vi "execute.vi"(8 "error in (no error)":errorcluster, 9 "image assembler in":refnum<class "GenericComponent.lvclass">, 10 "trajectory in":refnum<class "GenericComponent.lvclass">, 11 "AdapterMH111103TrajectoryToImageAssembler in":refnum<class "AdapterMH111103TrajectoryToImageAssembler.lvclass">) -> (0 "error out":errorcluster, 1 "image assembler out":refnum<class "GenericComponent.lvclass">, 2 "trajectory out":refnum<class "GenericComponent.lvclass">, 3 "AdapterMH111103TrajectoryToImageAssembler out":refnum<class "AdapterMH111103TrajectoryToImageAssembler.lvclass">)   [LabVIEW 2010, in "AdapterMH111103TrajectoryToImageAssembler.lvclass"]
uses:
  AdapterMH111103TrajectoryToImageAssembler.lvclass
  common/classes/GenericComponent/GenericComponent/GenericComponent.lvclass
  ImageAssembler/ImageAssemblerDL090211Frame/ImageAssemblerDL090211Frame/ImageAssemblerDL090211Frame.lvclass
  Trajectory/TrajectoryMG100122AODFrameScan/TrajectoryMG100122AODFrameScan/TrajectoryMG100122AODFrameScan.lvclass
  common/classes/Box/Box/Box.lvclass
  common/classes/SpaceVector/SpaceVector/SpaceVector.lvclass
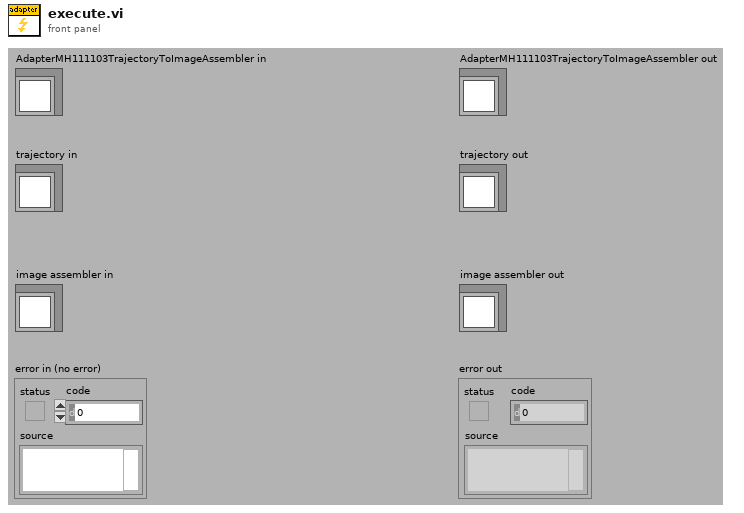
[diagram p1: front panel]
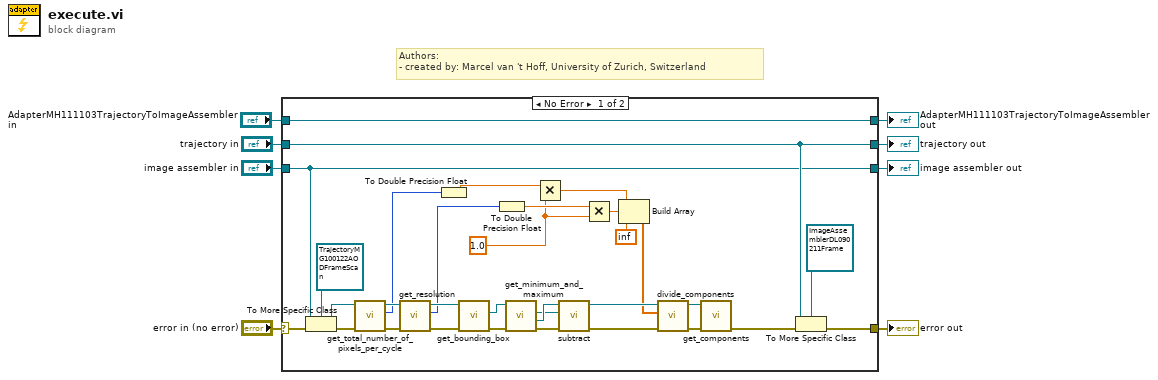
[diagram p0: block diagram]
diagram:
  # "Authors: \n- created by: Marcel van 't Hoff, University of Zurich, Switzerland"
  n1 = case shown="No Error" "error in (no error)" {
    selector: "error in (no error)" -> [w20 w43]
    tunnel: [w19 w43] -> w4
    tunnel: [w40 w44] -> w1
    tunnel: "AdapterMH111103TrajectoryToImageAssembler in" -> [w40 w44]
    tunnel: [w37 w42] -> w2
    tunnel: "trajectory in" -> [w37 w42]
    tunnel: [w9 w41] -> w3
    tunnel: "image assembler in" -> [w9 w41]
    frame No Error {
      w11 = 1.0
      n2 = To More Specific Class(target class=refnum<class "TrajectoryMG100122AODFrameScan.lvclass"> refnum ("TrajectoryMG100122AODFrameScan.lvclass"), reference=w9, error in=w20) -> (specific class reference=w36:refnum<class "TrajectoryMG100122AODFrameScan.lvclass">, error out=w33:errorcluster)
      n3 = call-dynamic "get_total_number_of_pixels_per_cycle.vi"("error in (no error)"=w33, "TrajectoryMG100122AODFrameScan in"=w36) -> ("error out"=w34:errorcluster, "total number of pixels per cycle"=w13:i32, "TrajectoryMG100122AODFrameScan out"=w35:refnum<class "TrajectoryMG100122AODFrameScan.lvclass">)  [unwired: 7 in]
      n4 = call-dynamic "get_resolution.vi"("error in (no error)"=w34, "TrajectoryMG100122AODFrameScan in"=w35) -> ("error out"=w22:errorcluster, "x resolution"=w12:i32, "TrajectoryMG100122AODFrameScan out"=w23:refnum<class "TrajectoryMG100122AODFrameScan.lvclass">)  [unwired: 6 in, 1 out]
      n5 = To Double Precision Float(number=w13) -> (double precision float=w15:dbl)
      n6 = call-dynamic "get_bounding_box.vi"("error in (no error)"=w22, "GenericTrajectory in"=w23) -> ("error out"=w24:errorcluster, "Box.lvclass"=w25:refnum<class "Box.lvclass">)  [unwired: 7 in, 1 out]
      n7 = To Double Precision Float(number=w12) -> (double precision float=w16:dbl)
      n8 = call "get_minimum_and_maximum.vi"("error in (no error)"=w24, "Box in"=w25) -> ("error out"=w26:errorcluster, "maximum"=w28:refnum<class "SpaceVector.lvclass">, "minimum"=w27:refnum<class "SpaceVector.lvclass">)  [unwired: 7 out]
      n9 = Multiply(x=w15, y=w11) -> (x*y=w17:dbl)
      n10 = call "subtract.vi"("error in (no error)"=w26, "subtrahend"=w27, "SpaceVector in"=w28) -> ("error out"=w29:errorcluster, "SpaceVector out"=w30:refnum<class "SpaceVector.lvclass">)  [unwired: 7 out]
      n11 = Multiply(x=w16, y=w11) -> (x*y=w18:dbl)
      n12 = Build Array(w17, w18, inf) -> (w10:dbl[])
      n13 = call "divide_components.vi"("error in (no error)"=w29, "divisors"=w10, "SpaceVector in"=w30) -> ("error out"=w31:errorcluster, "SpaceVector out"=w32:refnum<class "SpaceVector.lvclass">)  [unwired: 7 out]
      n14 = call "get_components.vi"("error in (no error)"=w31, "SpaceVector in"=w32) -> ("error out"=w21:errorcluster)  [unwired: 9 out]
      n15 = To More Specific Class(target class=refnum<class "ImageAssemblerDL090211Frame.lvclass"> refnum ("ImageAssemblerDL090211Frame.lvclass"), reference=w37, error in=w21) -> (error out=w19:errorcluster)  [unwired: 1 out]
    }
    frame Error {
    }
  }
  "error out" <- w4
  "AdapterMH111103TrajectoryToImageAssembler out" <- w1
  "trajectory out" <- w2
  "image assembler out" <- w3
